vi "Close.vi"(8 "error in":errorcluster, 11 "AO DAQmx DC CFG in":refnum<class "AO DAQmx DC CFG.lvclass">) -> (0 "error out":errorcluster, 3 "AO DAQmx DC CFG out":refnum<class "AO DAQmx DC CFG.lvclass">)   [LabVIEW 2024, in "AO DAQmx DC CFG.lvclass"]
uses:
  AO DAQmx DC CFG.lvclass
  AO DAQmx DC CFG.lvclass/AO DAQmx DC CFG.ctl
  DAQmx Base CFG/DAQmx Base CFG.lvclass
  Buffers/BufferWrites1SamDBL/BufferWrites1SamDBL.lvclass
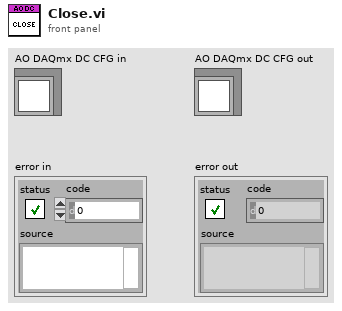
[diagram p1: front panel]
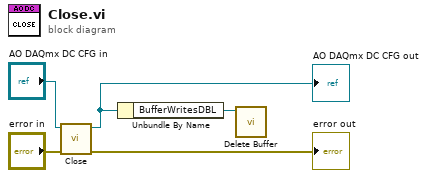
[diagram p0: block diagram]
diagram:
  n1 = call-parent "Close.vi"("error in"="error in", "DAQmx Base CFG in"="AO DAQmx DC CFG in") -> ("error out"=→"error out":errorcluster, "DAQmx Base CFG out"=w3:refnum<class "AO DAQmx DC CFG.lvclass">)  [unwired: 8 in]
  "AO DAQmx DC CFG out" <- w3
  n2 = Unbundle By Name(w3) -> ("BufferWritesDBL"=w2:refnum<class "BufferWrites1SamDBL.lvclass">)
  n3 = call-dynamic "Delete Buffer.vi"("BufferWrites1SamDBL in"=w2) -> ()  [unwired: 10 in, 1 out]
